vi "USBTC08GetSingleExample.vi"() -> ()   [LabVIEW 2010]
panel:
  out "?":dynamicdata(graph)
  in  "Units":enum16{"C°", "F°", "K°", "R°"}(ring)
  out "Unit Info":T1
  out "handle":i16
  out "error out":errorcluster
  in  "Channel Settings":T2={"Type # 1"=107, "Ch# 1"=TRUE, "Type # 2"=107, "Ch# 2"=FALSE, "Type # 3"=107, "Ch # 3"=FALSE, "Type # 4"=107, "Ch # 4"=FALSE, "Type # 5"=107, "Ch # 5"=FALSE, "Type # 6"=107, "Ch # 6"=FALSE, "Type # 7"=107, "Ch # 7"=FALSE, "Type # 8"=107, "Ch # 8"=FALSE, "CJC"=TRUE} {"Type # 8" items=["B"=98, "E"=101, "J"=106, "K"=107, "N"=110, "R"=114, "S"=115, "T"=116, "Voltage"=120]; "Type # 7" items=["B"=98, "E"=101, "J"=106, "K"=107, "N"=110, "R"=114, "S"=115, "T"=116, "Voltage"=120]; "Type # 6" items=["B"=98, "E"=101, "J"=106, "K"=107, "N"=110, "R"=114, "S"=115, "T"=116, "Voltage"=120]; "Type # 5" items=["B"=98, "E"=101, "J"=106, "K"=107, "N"=110, "R"=114, "S"=115, "T"=116, "Voltage"=120]; "Type # 4" items=["B"=98, "E"=101, "J"=106, "K"=107, "N"=110, "R"=114, "S"=115, "T"=116, "Voltage"=120]; "Type # 3" items=["B"=98, "E"=101, "J"=106, "K"=107, "N"=110, "R"=114, "S"=115, "T"=116, "Voltage"=120]; "Type # 2" items=["B"=98, "E"=101, "J"=106, "K"=107, "N"=110, "R"=114, "S"=115, "T"=116, "Voltage"=120]; "Type # 1" items=["B"=98, "E"=101, "J"=106, "K"=107, "N"=110, "R"=114, "S"=115, "T"=116, "Voltage"=120]}
  in  "error in (no error)":errorcluster
  in  "Mains Frequency":i16(ring) items=["50 Hz", "60 Hz"]
  in  "stop":bool
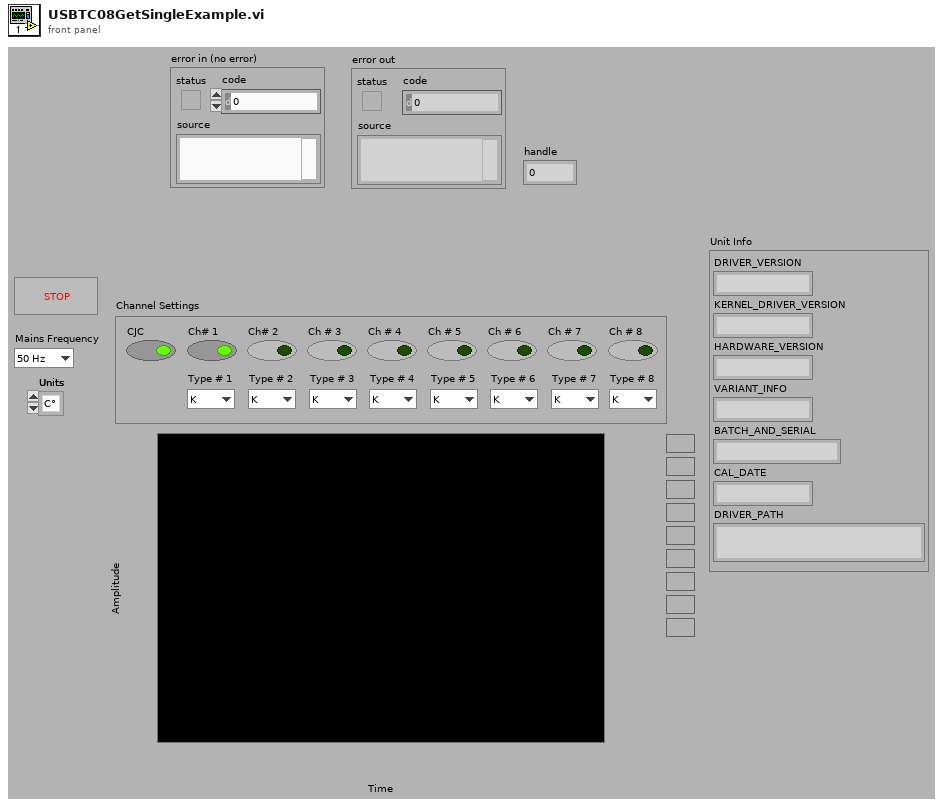
[diagram p1: front panel]
types:
  T1 = cluster{"DRIVER_VERSION":string, "KERNEL_DRIVER_VERSION":string, "HARDWARE_VERSION":string, "VARIANT_INFO":string, "BATCH_AND_SERIAL":string, "CAL_DATE":string, "DRIVER_PATH":string, "[7]":string, "[8]":string, "[9]":string, "[10]":string, "[11]":string, "[12]":string, "[13]":string, "[14]":string}
  T2 = cluster{"Type # 1":i16, "Ch# 1":bool, "Type # 2":i16, "Ch# 2":bool, "Type # 3":i16, "Ch # 3":bool, "Type # 4":i16, "Ch # 4":bool, "Type # 5":i16, "Ch # 5":bool, "Type # 6":i16, "Ch # 6":bool, "Type # 7":i16, "Ch # 7":bool, "Type # 8":i16, "Ch # 8":bool, "CJC":bool}
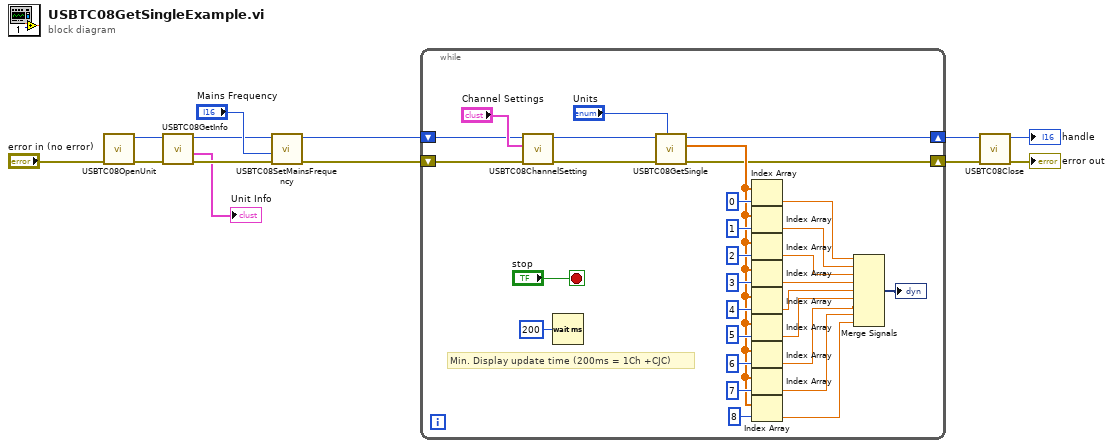
[diagram p0: block diagram]
diagram:
  n1 = call "USBTC08OpenUnit.vi"("error in (no error)"="error in (no error)") -> ("error out"=w7:errorcluster, "Handle out"=w6:i16)  [unwired: 9 in]
  n2 = call "USBTC08GetInfo.vi"("error in (no error)"=w7, "Handle in"=w6) -> ("error out"=w4:errorcluster, "Unit Info"=→"Unit Info":T1, "Handle out"=w5:i16)  [unwired: 7 in]
  n3 = call "USBTC08SetMainsFrequency.vi"("error in (no error)"=w4, "Mains Frequency"="Mains Frequency", "Handle in"=w5) -> ("error out"=w2:errorcluster, "Handle out"=w1:i16)  [unwired: 7 in]
  n4 = while {
    shift-right: [w20] -> w9
    shift-left: w1 -> [w25]
    shift-right: [w19] -> w8
    shift-left: w2 -> [w26]
    stop <- "stop" stop-if-true
    # "Min. Display update time (200ms = 1Ch +CJC)"
    n5 = call "USBTC08ChannelSetting.vi"("error in (no error)"=w26, "Channel Settings"="Channel Settings", "Handle In"=w25) -> ("error out"=w23:errorcluster, "Handle out"=w24:i16)  [unwired: 6 in, 1 out]
    n6 = Wait (ms)(milliseconds to wait=u32 200) -> ()  [unwired: 1 out]
    n7 = call "USBTC08GetSingle.vi"("Units"="Units", "error in (no error)"=w23, "Handle in"=w24) -> ("error out"=w19:errorcluster, "Array out"=w21:sgl[], "Handle out"=w20:i16)  [unwired: 5 in, 1 out]
    n8 = Index Array(array=w21, index=i16 0) -> (element=w33:sgl)
    n9 = Index Array(array=w21, index=i16 1) -> (element=w30:sgl)
    n10 = Index Array(array=w21, index=i16 2) -> (element=w32:sgl)
    n11 = Index Array(array=w21, index=i16 3) -> (element=w31:sgl)
    n12 = Index Array(array=w21, index=4) -> (element=w18:sgl)
    n13 = Index Array(array=w21, index=i16 5) -> (element=w17:sgl)
    n14 = Index Array(array=w21, index=6) -> (element=w16:sgl)
    n15 = Index Array(array=w21, index=i16 7) -> (element=w15:sgl)
    n16 = Index Array(array=w21, index=i16 8) -> (element=w14:sgl)
    n17 = Merge Signals(w33, w30, w32, w31, w18, w17, w16, w15, w14) -> (→"?":dynamicdata)
  }
  n18 = call "USBTC08Close.vi"("error in (no error)"=w8, "Handle in"=w9) -> ("error out"=→"error out":errorcluster, "handle"=→"handle":i16)  [unwired: 8 in]
